vi "AutoDrive.vi"(9 "Angle PID gains":T1={"proportional gain (Kc)"=1.0, "integral time (Ti, min)"=0.01, "derivative time (Td, min)"=0.0} {"derivative time (Td, min)" format="%.3f"; "integral time (Ti, min)" format="%.3f"; "proportional gain (Kc)" format="%.3f"}, 10 "PID gains":T1={"proportional gain (Kc)"=3.3, "integral time (Ti, min)"=0.5, "derivative time (Td, min)"=0.001} {"derivative time (Td, min)" format="%.3f"; "integral time (Ti, min)" format="%.3f"; "proportional gain (Kc)" format="%.3f"}, 11 "Input":dbl format="%#_13g") -> (0 "error out":errorcluster, 1 "Distance":cluster{"Rate":dbl, "Rate":dbl})   [LabVIEW 2013]
uses:
  <vilib>/Rock Robotics/WPI/RobotDrive/WPI_RobotDriveGetSetRefNum.vi
  <vilib>/addons/control/pid/pid.llb/PID Control Input Filter (DBL).vi
  <vilib>/addons/control/pid/pid.llb/PID (DBL).vi
  <vilib>/Rock Robotics/WPI/RobotDrive/WPI_RobotDriveArcadeDrive_Standard(NoSaturation).vi
  <vilib>/addons/control/pid/NI_PID_pid.lvlib
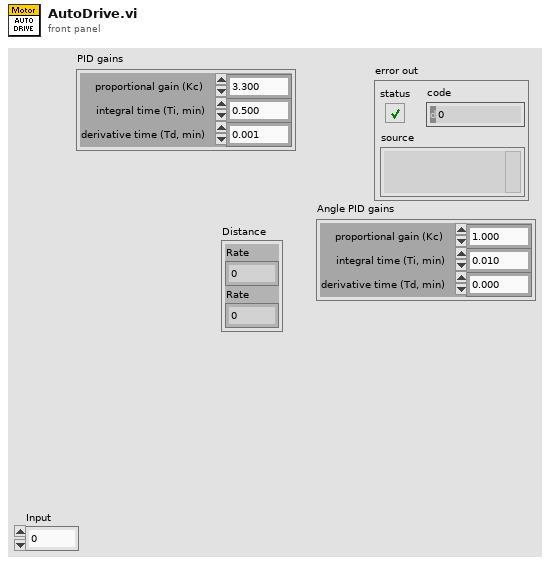
[diagram p1: front panel]
types:
  T1 = cluster{"proportional gain (Kc)":dbl, "integral time (Ti, min)":dbl, "derivative time (Td, min)":dbl}
  T2 = typedef "WPI_RobotDriveDevRef.ctl" = cluster{"DevStatus":errorcluster, "Motors[]":T3[], "Square Inputs":bool, "Max Output":dbl, "Isochronous":bool}
  T3 = typedef "WPI_MotorControlDeviceRef.ctl" = cluster{"DeviceStatus":errorcluster, "Type":enum16{"PWM", "CAN"}, "PWM":cluster{"Digital Module":T4, "PWM Channel":T5, "DeadBand":T6}, "CAN":cluster{"Device Number":u8, "Control Mode":T7, "Semaphore":T8, "Max Vout":dbl}, "Invert":bool, "TransformRef":T9, "InvTransformRef":T9}
  T4 = typedef "FPGA_TypedefDigitalModule.ctl" = enum16{"Digital Module 1", "Digital Module 2"}
  T5 = typedef "FPGA_DIOPWMChannel.ctl" = enum8{"PWM 1", "PWM 2", "PWM 3", "PWM 4", "PWM 5", "PWM 6", "PWM 7", "PWM 8", "PWM 9", "PWM 10", "Invalid"}
  T6 = typedef "WPI_PWMDeadband.ctl" = cluster{"Name":string, "maxPositivePwm":i32, "minPositivePwm":i32, "centerPwm":i32, "maxNegativePwm":i32, "minNegativePwm":i32, "angularRange":u16}
  T7 = typedef "WPI_CANJaguar_ControlMode.ctl" = enum8{"Percent VBus", "Current", "Speed", "Position", "Voltage"}
  T8 = typedef "Semaphore RefNum" = refnum<k1>
  T9 = typedef "WPI_PWMTransform_ConPane.ctl" = refnum<vi>
  T10 = typedef "WPI_EncoderDevRef.ctl" = cluster{"DevStatus":errorcluster, "EncoderIndex":T11, "CounterIndex":T12, "DistancePerCount":dbl, "Decoding Type":T13}
  T11 = typedef "FPGA_EncoderIdx.ctl" = enum8{"Enc 0", "Enc 1", "Enc 2", "Enc 3", "Invalid"}
  T12 = typedef "FPGA_CounterCtrSystemIndex.ctl" = enum8{"Ctr 0", "Ctr 1", "Ctr 2", "Ctr 3", "Ctr 4", "Ctr 5", "Ctr 6", "Ctr 7", "Invalid"}
  T13 = typedef "WPI_EncoderType.ctl" = enum16{"1x", "2x", "4x"}
  T14 = typedef "WPI_CounterDevRef.ctl" = cluster{"DevStatus":errorcluster, "CntIndex":T12}
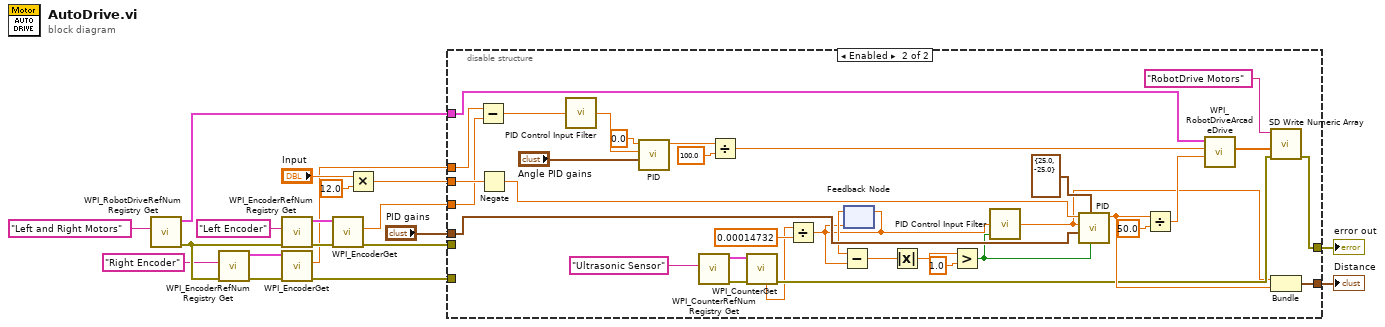
[diagram p0: block diagram]
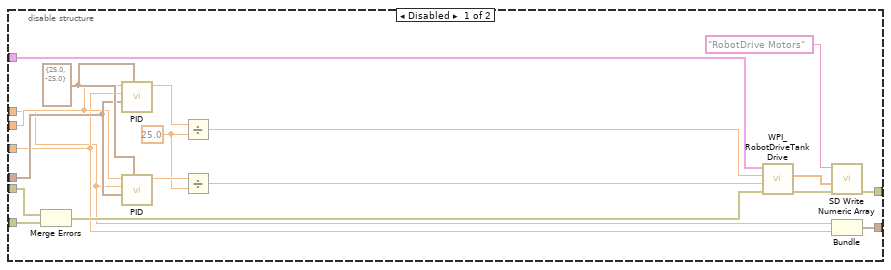
[diagram p2: hidden frame]
diagram:
  n1 = call <vilib>:"WPI_RobotDriveRefNum Registry Get.vi"("refnum name"="Left and Right Motors") -> ("error out"=w14:errorcluster, "RobotDriveDevRef"=w2:T2)  [unwired: 9 in]
  n2 = call <vilib>:"WPI_EncoderRefNum Registry Get.vi"("error in (no error)"=w14, "refnum name"="Right Encoder") -> ("error out"=w11:errorcluster, "EncoderDevRef"=w12:T10)  [unwired: 8 in]
  n3 = call <vilib>:"WPI_EncoderRefNum Registry Get.vi"("error in (no error)"=w14, "refnum name"="Left Encoder") -> ("error out"=w9:errorcluster, "EncoderDevRef"=w10:T10)  [unwired: 8 in]
  n4 = call <vilib>:"WPI_EncoderGet.vi"("error in (no error)"=w11, "EncoderDevRef"=w12) -> ("error out"=w4:errorcluster, "Distance"=w5:dbl)  [unwired: 4 in, 4 out]
  n5 = call <vilib>:"WPI_EncoderGet.vi"("error in (no error)"=w9, "EncoderDevRef"=w10) -> ("error out"=w3:errorcluster, "Distance"=w6:dbl)  [unwired: 4 in, 4 out]
  n6 = Multiply(x="Input", y=12.0) -> (x*y=w7:dbl)
  n7 = disable-structure shown="Enabled" {
    disable-tunnel: "PID gains" -> [w27 w65]
    disable-tunnel: [w28 w66] -> w18
    disable-tunnel: w7 -> [w26 w64]
    disable-tunnel: w6 -> [w25 w51]
    disable-tunnel: w5 -> [w24 w52]
    disable-tunnel: w4 -> [w23 _]
    disable-tunnel: w3 -> [w22 _]
    disable-tunnel: w2 -> [w21 w63]
    disable-tunnel: [w20 w55] -> w1
    frame Disabled {
      w29 = cluster{"output high":dbl, "output low":dbl} {"output high"=25.0, "output low"=-25.0} ("output range")
      w30 = 25.0 ("y")
      n8 = Merge Errors(w22, w23) -> (w38:errorcluster)
      n9 = call-poly <vilib>:"PID.vi"("output range"=w29, "PID gains"=w27, "process variable"=w25, "setpoint"=w26) -> ("output"=w31:dbl)  [unwired: 6 in, 1 out]
      n10 = call-poly <vilib>:"PID.vi"("output range"=w29, "PID gains"=w27, "process variable"=w24, "setpoint"=w26) -> ("output"=w32:dbl)  [unwired: 6 in, 1 out]
      n11 = Divide(x=w31, y=w30) -> (x/y=w33:dbl)
      n12 = Divide(x=w32, y=w30) -> (x/y=w34:dbl)
      n13 = call <vilib>:"WPI_RobotDriveTankDrive.vi"("error in (no error)"=w38, "Right axis value"=w34, "Left axis value"=w33, "RobotDriveDevRef"=w21) -> ("error out"=w37:errorcluster, "Motor Values"=w36:dbl[])  [unwired: 5 in, 1 out]
      n14 = call <vilib>:"SD Write Numeric Array.vi"("error in"=w37, "Numeric Array"=w36, "Name"="RobotDrive Motors") -> ("error out"=w28:errorcluster)  [unwired: 7 in, 1 out]
      n15 = Bundle("Distance"=w24, "Distance"=w25) -> (w20:cluster{"Distance":dbl, "Distance":dbl})  [unwired: 1 in]
    }
    frame Enabled {
      n16 = Subtract(x=w52, y=w51) -> (x-y=w60:dbl)
      n17 = Negate(x=w64) -> (-x=w54:dbl)
      n18 = call-poly <vilib>:"PID Control Input Filter.vi"("input"=w60) -> ("output"=w49:dbl)  [unwired: 4 in]
      n19 = call-poly <vilib>:"PID.vi"("PID gains"="Angle PID gains", "process variable"=w49, "setpoint"=0.0) -> ("output"=w57:dbl)  [unwired: 7 in, 1 out]
      n20 = call <vilib>:"WPI_CounterRefNum Registry Get.vi"("refnum name"="Ultrasonic Sensor") -> ("error out"=w68:errorcluster, "CounterDevRef"=w69:T14)  [unwired: 9 in]
      n21 = Divide(x=w57, y=100.0) -> (x/y=w53:dbl)
      n22 = call <vilib>:"WPI_CounterGet.vi"("error in (no error)"=w68, "CounterDevRef in"=w69) -> ("error out"=w47:errorcluster, "Period (sec)"=w46:dbl)  [unwired: 4 in, 4 out]
      n23 = Divide(x=w46, y=0.00014732) -> (x/y=w39:dbl)
      n24 = feedback-in #1(w39) -> ()
      n25 = feedback #1(w39) -> (w40:dbl)
      n26 = Subtract(x=w40, y=w39) -> (x-y=w41:dbl)
      n27 = Absolute Value(x=w41) -> (abs(x)=w45:dbl)
      n28 = Greater?(x=w45, y=1.0) -> (0:w42:bool)
      n29 = call-poly <vilib>:"PID Control Input Filter.vi"("reinitialize? (F)"=w42, "input"=w39) -> ("output"=w43:dbl)  [unwired: 3 in]
      n30 = call-poly <vilib>:"PID.vi"("reinitialize? (F)"=w42, "output range"=cluster{"output high":dbl, "output low":dbl} {"output high"=25.0, "output low"=-25.0}, "PID gains"=w65, "process variable"=w43, "setpoint"=w54) -> ("output"=w48:dbl)  [unwired: 5 in, 1 out]
      n31 = Divide(x=w48, y=50.0) -> (x/y=w50:dbl)
      n32 = call-poly <vilib>:"WPI_RobotDriveArcadeDrive.vi"("Y axis value"=w50, "X axis value"=w53, "RobotDriveDevRef"=w63) -> ("Motor Values"=w71:dbl[])  [unwired: 6 in, 2 out]
      n33 = call <vilib>:"SD Write Numeric Array.vi"("error in"=w47, "Numeric Array"=w71, "Name"="RobotDrive Motors") -> ("error out"=w66:errorcluster)  [unwired: 7 in, 1 out]
      n34 = Bundle("output"=w43, "output"=w48) -> (w55:cluster{"output":dbl, "output":dbl})  [unwired: 1 in]
    }
  }
  "error out" <- w18
  "Distance" <- w1
